vi "MultiChannelFeedback_test_no_before (FPGA).vi"() -> ()   [LabVIEW 2016]
doc: "This VI will read single point values from 4 channels of a R Series board at a specified rate."
uses:
  <vilib>/rvi/Emulation/niFpgaGetClockAttributes.vi
  <vilib>/rvi/Emulation/niFpgaSctlEmulationGetInTimedLoop.vi
  <vilib>/rvi/Emulation/niFpgaEmulationReportErrorSimple.vi
  <vilib>/rvi/Emulation/niFpgaProcessEmulError.vi
  <vilib>/rvi/eio/common/nirviEmuTemplateMethod_errors.vi
  <vilib>/rvi/Emulation/niFpgaCriticalErrorInLSC.vi
  <vilib>/rvi/Memory/Memory_Emulation/nirvimemoryFastEmulation.vi
  <vilib>/rvi/Memory/Memory_Emulation/nirvimemoryEmulation.vi
  <vilib>/rvi/Emulation/niFpgaEmulationIsFPGAContextNoSignature.vi
  <vilib>/rvi/DataTransferAndStorage/Container/Common/niFpgaContainerGetUniqueNameForEmu.vi
  <vilib>/rvi/errors/nirviReportUnexpectedCaseInternalError (U32).vi
  <vilib>/rvi/Memory/Memory_Emulation/niFpgaMemoryEmulationCacheClearOnFirstRun.vi
  <vilib>/rvi/Memory/Memory_Emulation/nirvimemoryEmulationManagerCache_MakeExclusive.vi
  <vilib>/rvi/Memory/Memory_Emulation/niFpgaMemoryEmulationValidateCache.vi
  <vilib>/rvi/Memory/Memory_Emulation/nirvimemoryEmulationManagerCache_InsertValue.vi
  <vilib>/Utility/error.llb/Clear Errors.vi
  <vilib>/rvi/Memory/Memory_Emulation/nirvimemoryEmulationManagerCache_ReleaseExclusive.vi
  <vilib>/rvi/Memory/Memory_Emulation/nirvimemoryEmulationManagerCache_GetValue.vi
  <vilib>/rvi/Memory/Memory_Emulation/nirvimemoryEmulationManagerCache_SetValue.vi
  <vilib>/rvi/Emulation/niFpgaSctlEmulationResourceMgr.vi
  <vilib>/eio/EIONode/EIONode.xnode
  <vilib>/rvi/DataTransferAndStorage/Container/XNode/niFpgaContainer.xnode
  <vilib>/rvi/FXPMathLib/FxpInterpret/XNode/nifxpmath_Interpret.xnode
panel:
  in  "final filter coeff X":i32[](array[numeric])=[-955995012, 2025731616, 1001305, -1023351008, 2092954700, 1034533]
  in  "final filter coeff Y":i32[](array[numeric])=[-955995012, 2025731616, 1001305, -1023351008, 2092954700, 1034533]
  in  "final filter coeff Z":i32[](array[numeric])=[-955995012, 2025731616, 1001305, -1023351008, 2092954700, 1034533]
  in  "LP Coeff Z":i32[](array[numeric])=[1008310688, 32715568]
  in  "LP Coeff X":i32[](array[numeric])=[1008310688, 32715568]
  in  "LP Coeff Y":i32[](array[numeric])=[1008310688, 32715568]
  in  "LP Coeff band X":i32[](array[numeric])=[-955995012, 2025731616, 1001305, -1023351008, 2092954700, 1034533]
  in  "HP Coeff band X":i32[](array[numeric])=[-850883994, 1909449570, 958518847, -975456236, 2033039520, 1020559395]
  in  "dg band X":fxp<+/-,24,12>
  in  "HP Coeff X":i32[](array[numeric])=[946630756, 1010186290]
  out "tot_fb X plot":i16
  in  "DC offset X":i16
  out "fb X plot":i16
  in  "ig X":fxp<+/-,24,6>
  in  "Lower lim X":fxp<+/-,16,16>
  in  "Upper lim X":fxp<+/-,16,16>
  in  "dg X":fxp<+/-,24,12>
  in  "pg X":fxp<+/-,24,12>
  out "AI X plot":i16
  in  "X Setpoint":i16
  in  "LP Coeff band Y":i32[](array[numeric])=[-955995012, 2025731616, 1001305, -1023351008, 2092954700, 1034533]
  in  "HP Coeff band Y":i32[](array[numeric])=[-850883994, 1909449570, 958518847, -975456236, 2033039520, 1020559395]
  in  "dg band Y":fxp<+/-,24,12>
  in  "HP Coeff Y":i32[](array[numeric])=[946630756, 1010186290]
  out "tot_fb Y plot":i16
  in  "DC offset Y":i16
  out "fb Y plot":i16
  in  "ig Y":fxp<+/-,24,6>
  in  "Lower lim Y":fxp<+/-,16,16>
  in  "Upper lim Y":fxp<+/-,16,16>
  in  "dg Y":fxp<+/-,24,12>
  in  "pg Y":fxp<+/-,24,12>
  out "AI Y plot":i16
  in  "Y Setpoint":i16
  in  "EOM_offset":i16
  in  "EOM_seed":u32=4294967295 caption="seed"
  in  "EOM reset":bool caption="reset"
  in  "EOM_threshold":i16
  in  "EOM_amplitude":i16
  in  "LP Coeff band Z":i32[](array[numeric])=[-955995012, 2025731616, 1001305, -1023351008, 2092954700, 1034533]
  in  "HP Coeff band Z":i32[](array[numeric])=[-850883994, 1909449570, 958518847, -975456236, 2033039520, 1020559395]
  in  "dg band Z":fxp<+/-,24,12>
  in  "data_buffer3":i16
  in  "Arb gain (ch2)":fxp<+/-,24,12>=0.5 caption="RMS"
  in  "HP Coeff Z":i32[](array[numeric])=[946630756, 1010186290]
  out "tot_fb Z plot":i16
  in  "DC offset Z":i16
  out "fb Z plot":i16
  in  "ig Z":fxp<+/-,24,6>
  out "written_address":u32
  in  "ready_to_write":bool
  in  "Arb steps per cycle":u16
  in  "data_buffer2":i16
  in  "data_buffer_1":i16
  in  "write_address":u16
  in  "Arb gain (ch1)":fxp<+/-,24,12>=0.5 caption="RMS"
  in  "Arb gain (ch0)":fxp<+/-,24,12>=0.5 caption="RMS"
  in  "Lower lim Z":fxp<+/-,16,16>
  in  "Upper lim Z":fxp<+/-,16,16>
  in  "dg Z":fxp<+/-,24,12>
  in  "pg Z":fxp<+/-,24,12>
  out "AI Z plot":i16
  in  "Z Setpoint":i16
  in  "Count(uSec)":u32
  out "FPGA Error Out":errorcluster
  in  "Stop":bool
  # "test"
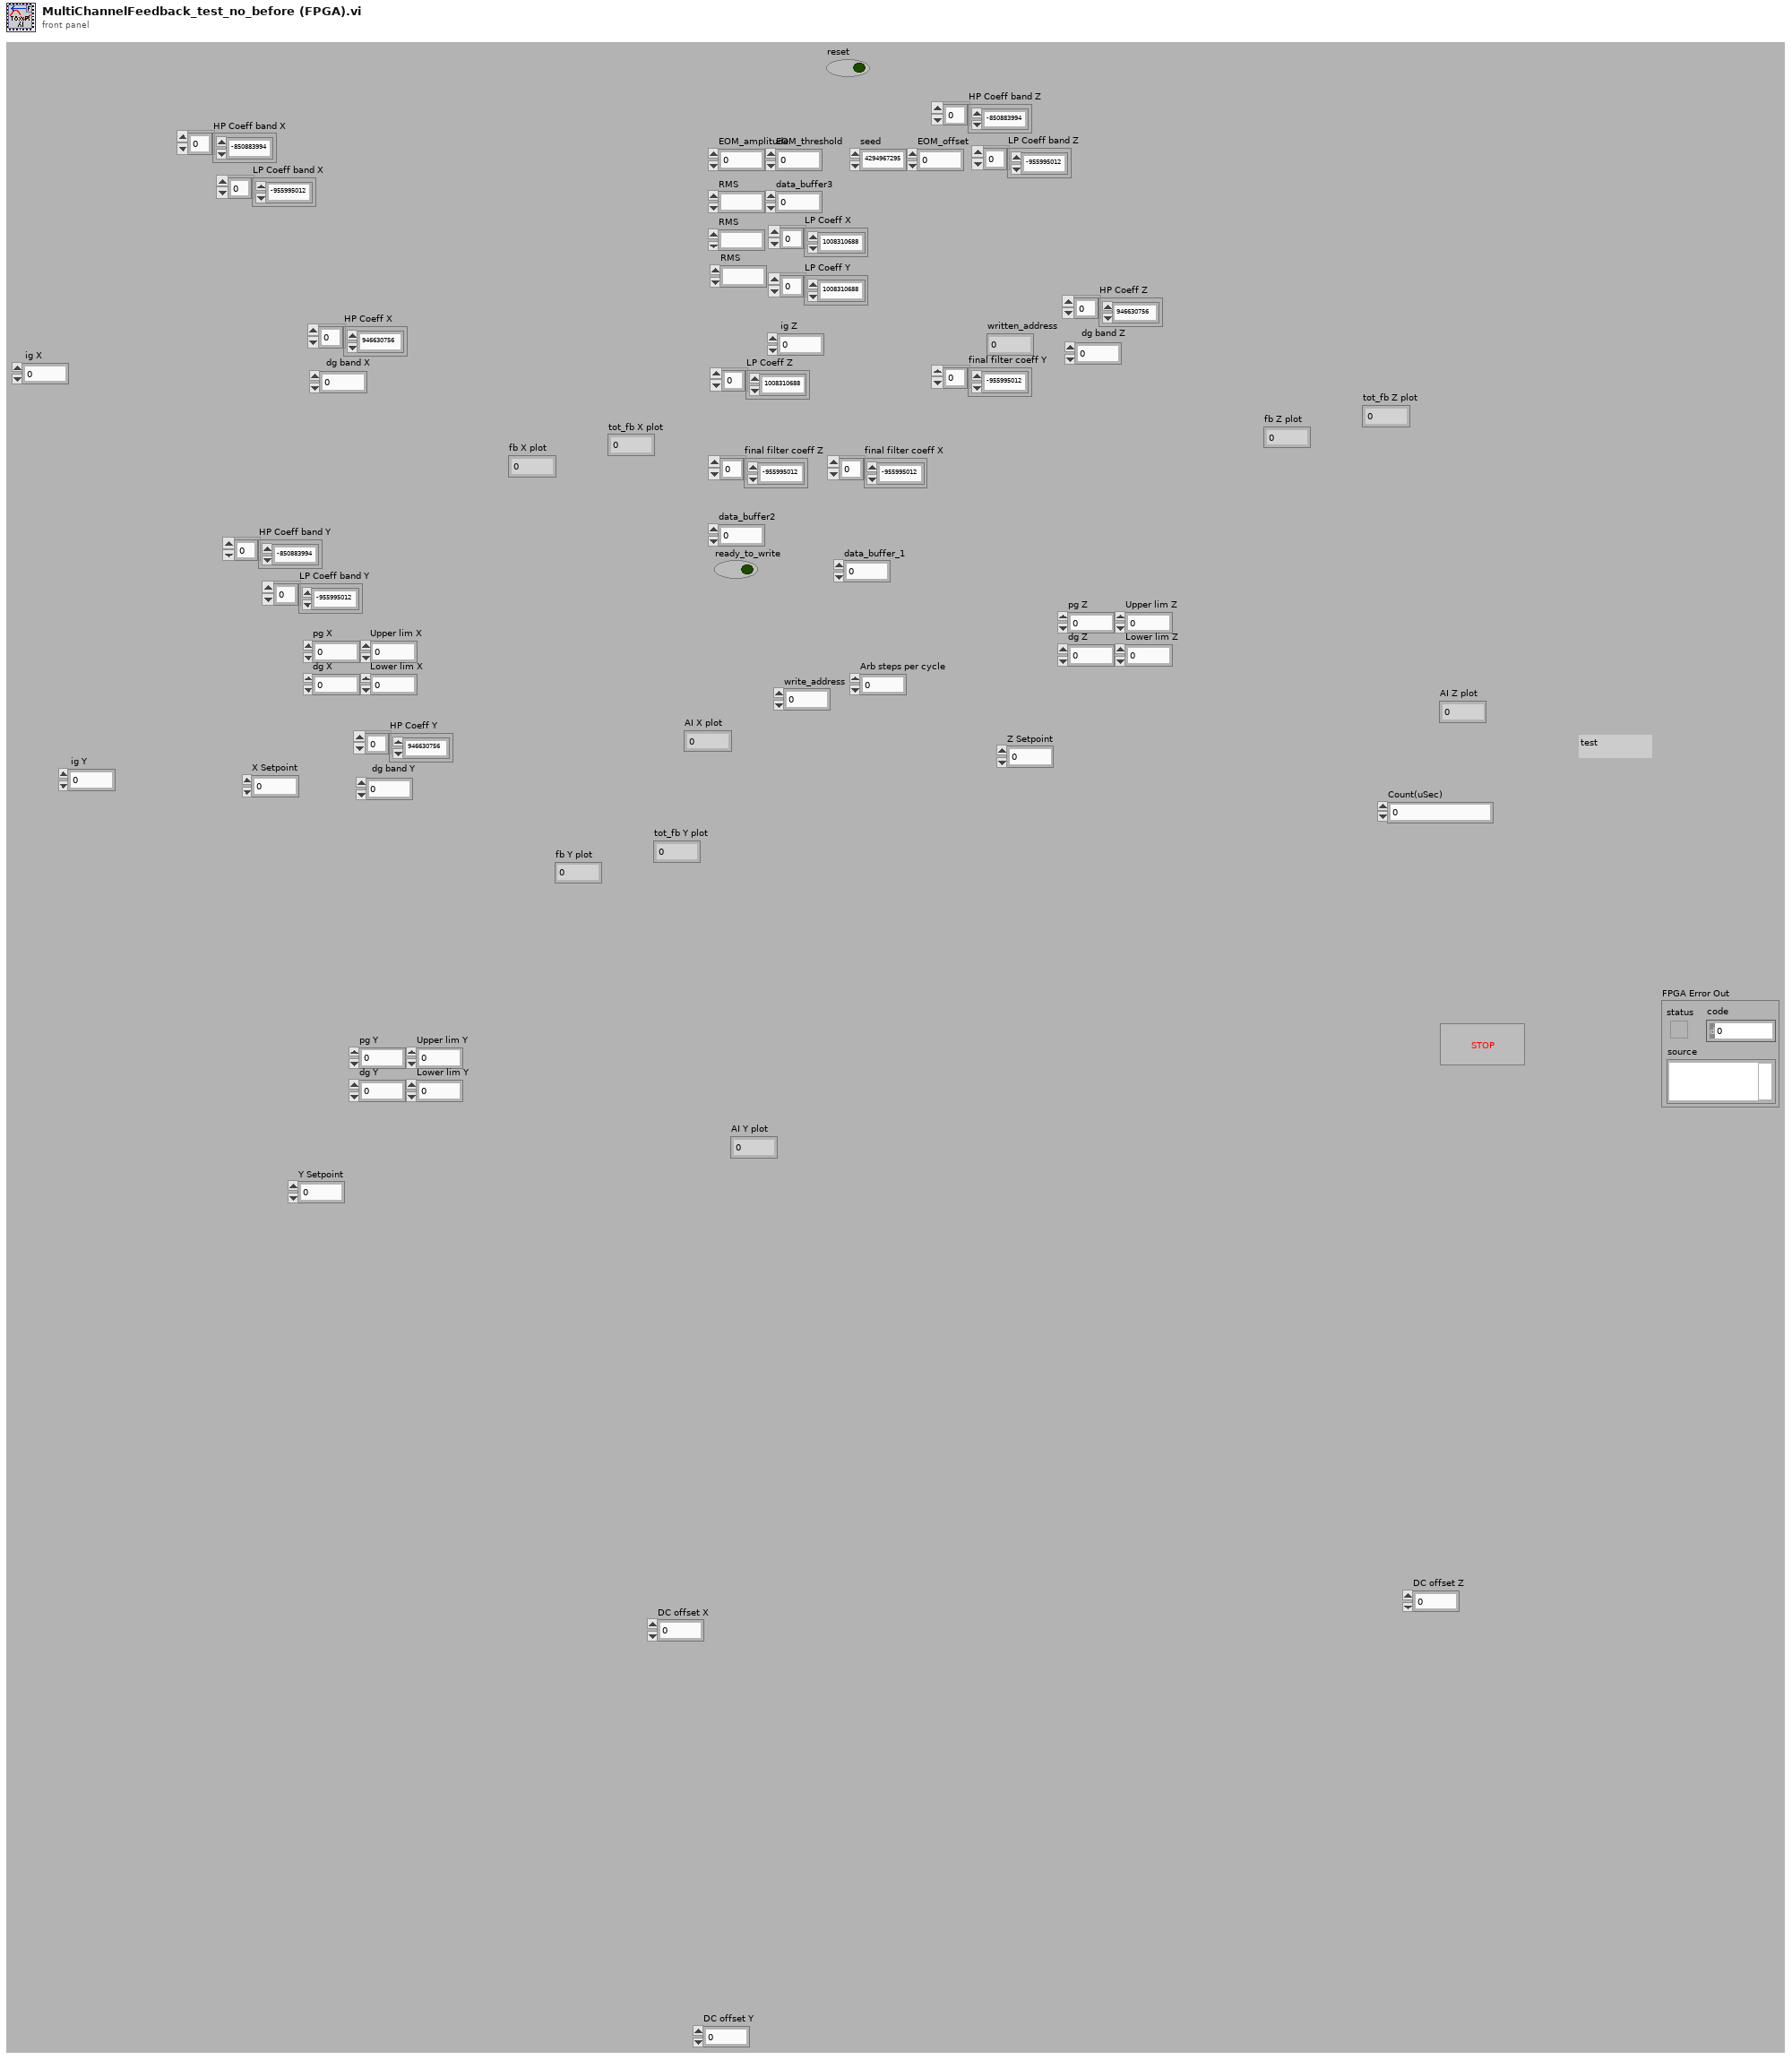
[diagram p1: front panel]
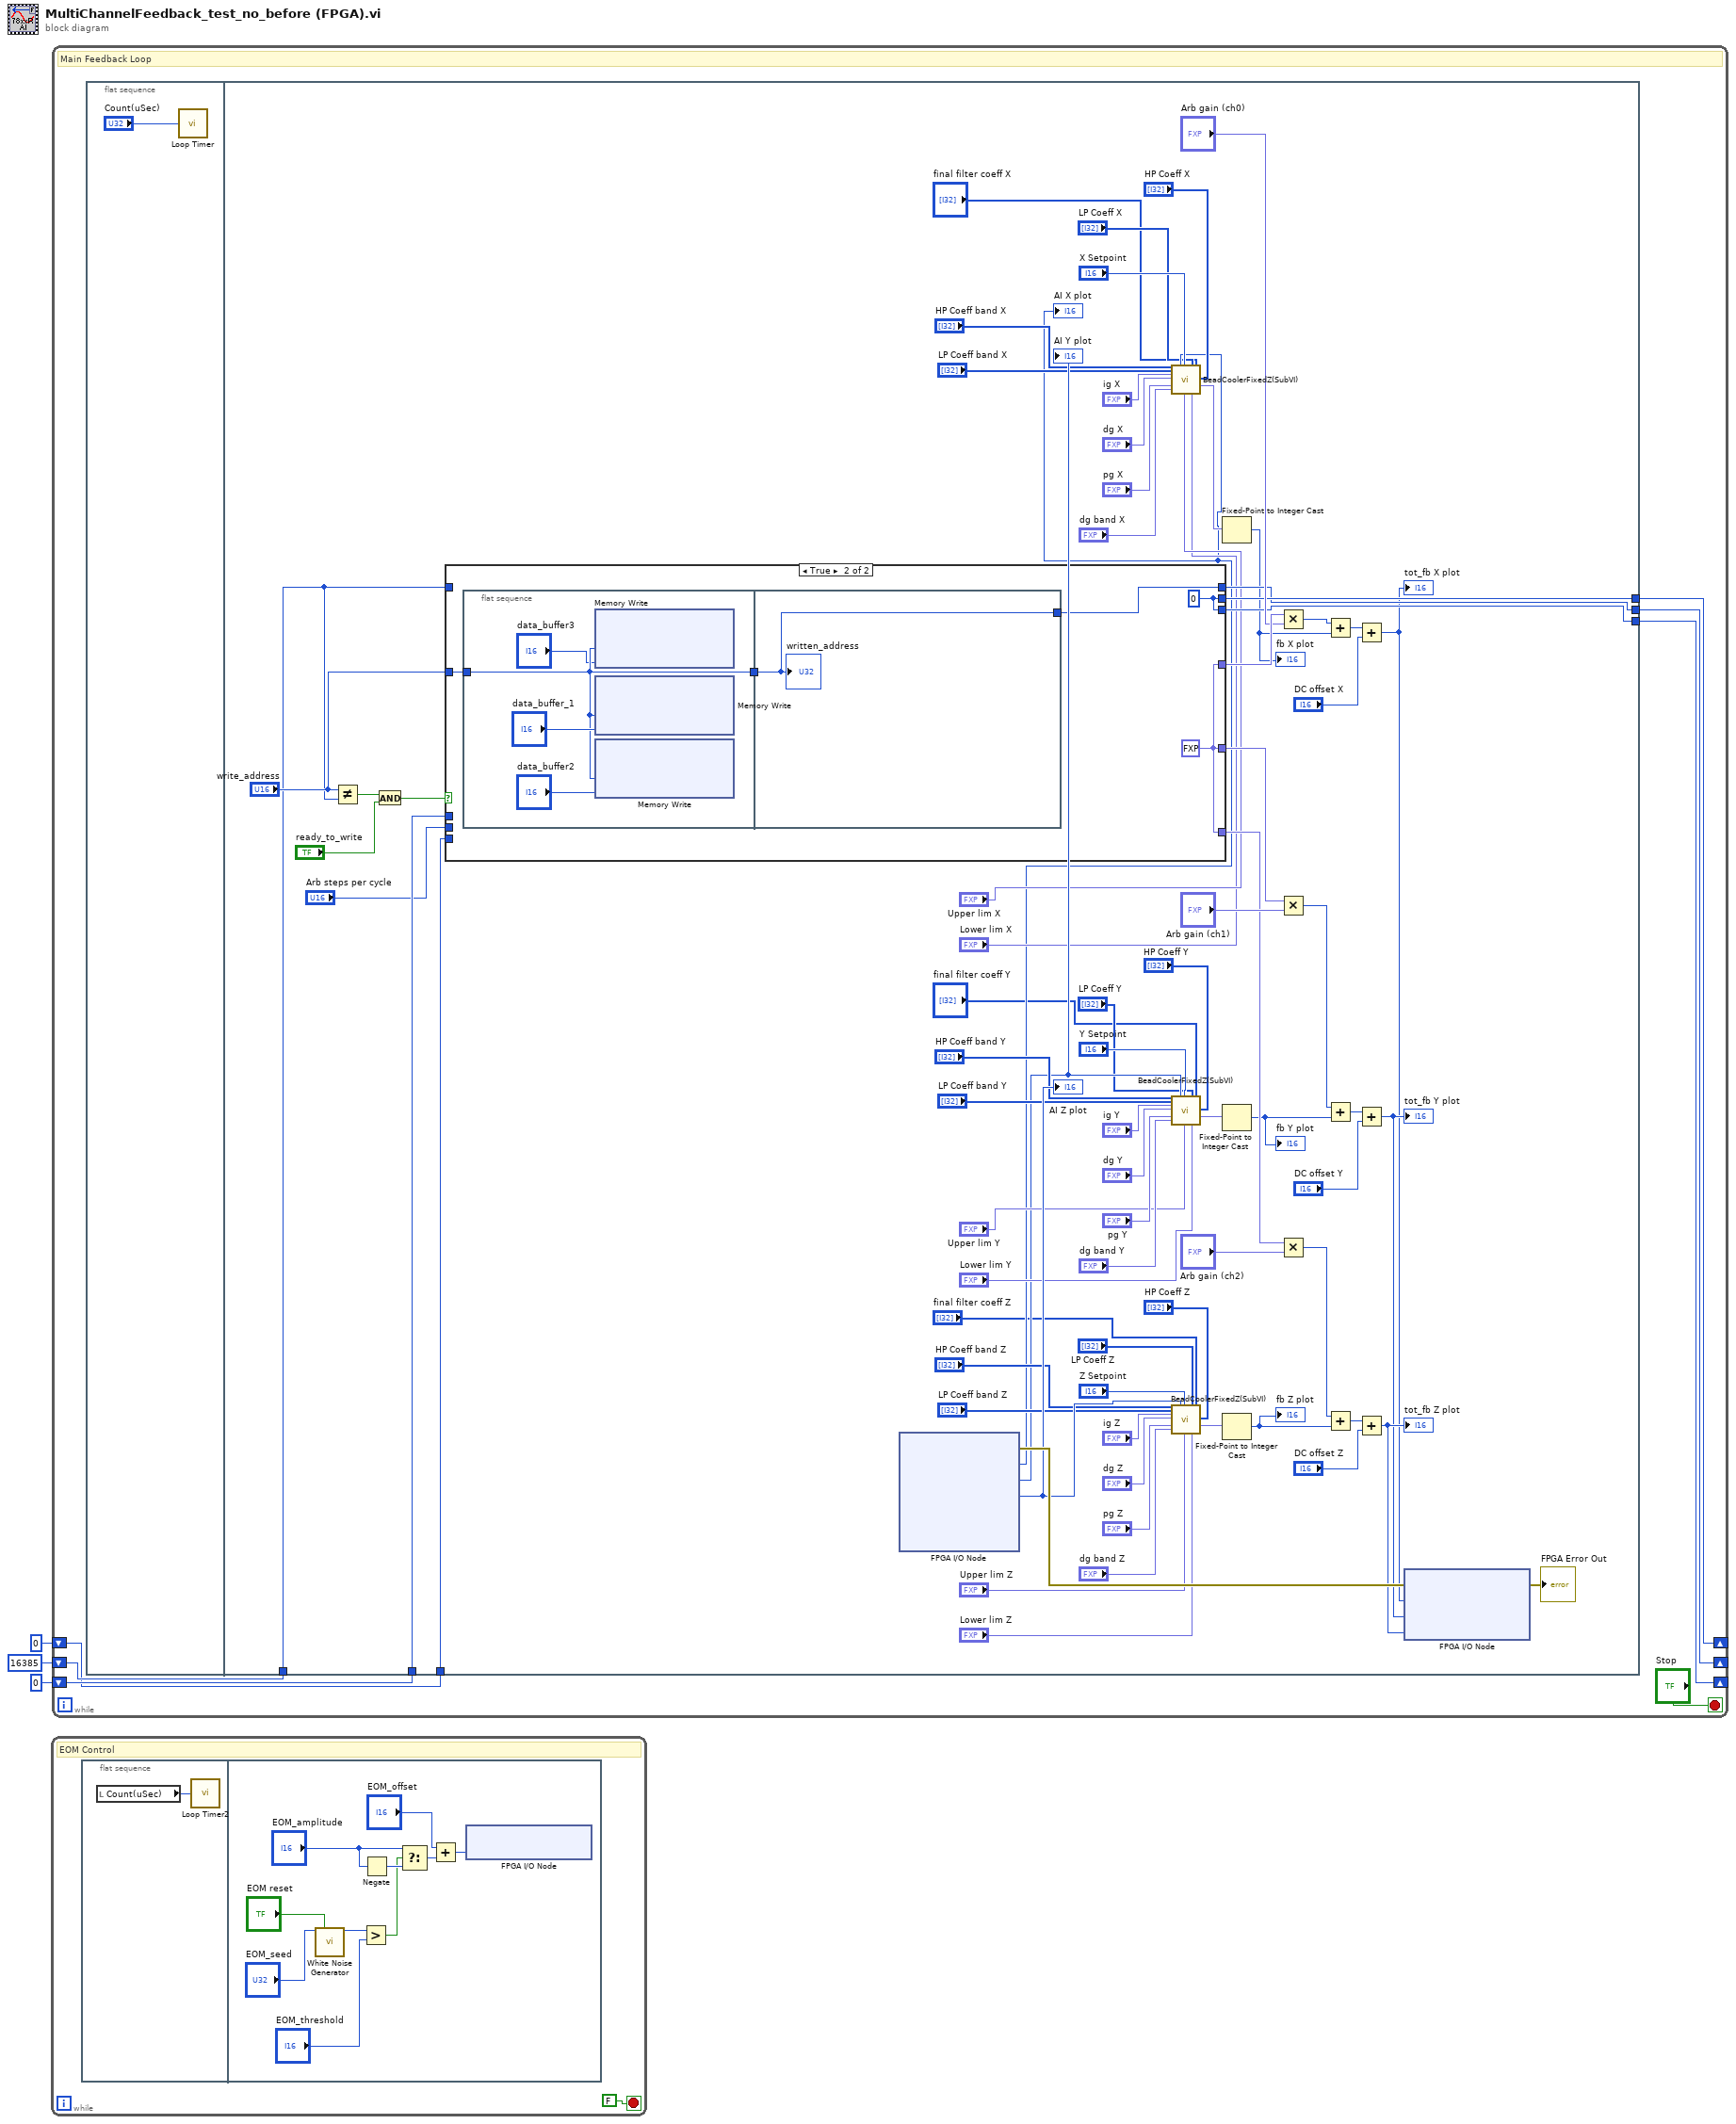
[diagram p0: block diagram]
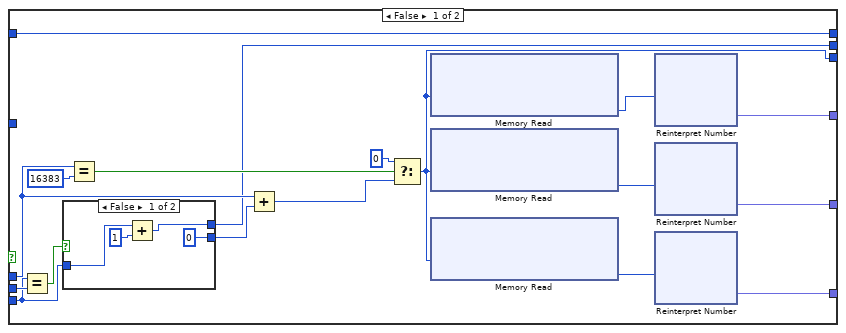
[diagram p2: hidden frame]
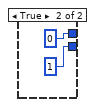
[diagram p3: hidden frame]
diagram:
  n1 = while {
    stop <- FALSE stop-if-true
    # "EOM Control"
    n2 = flat-sequence {
      frame #0 {
        n3 = local read "Count(uSec)"() -> (w5:u32)
        n4 = call "Loop Timer2"("Count(uSec)"=w5) -> ()  [unwired: 1 out]
      }
      frame #1 {
        n5 = call "White Noise Generator"("seed"="EOM_seed", "reset"="EOM reset") -> ("white noise out"=w7:i16)  [unwired: 13 in]
        n6 = Greater?(x=w7, y="EOM_threshold") -> (0:w9:bool)
        n7 = Negate(x="EOM_amplitude") -> (-x=w11:i16)
        n8 = Select(t="EOM_amplitude", s=w9, f=w11) -> (s? t:f=w14:i16)
        n9 = Add(x="EOM_offset", y=w14) -> (x+y=w6:i16)
        n10 = xnode "FPGA I/O Node"("Connector0/AO3"=w6) -> ()  [unwired: 1 in, 1 out]
      }
    }
  }
  n11 = while {
    shift-right: [w21] -> _
    shift-left: u16 0 ("t") -> [w20]
    shift-right: [w19] -> _
    shift-left: u16 0 ("t") -> [w16]
    shift-right: [w18] -> _
    shift-left: u32 16385 ("write_address") -> [w17]
    stop <- "Stop" stop-if-true
    # "Main Feedback Loop"
    n12 = flat-sequence {
      tunnel: [w92] -> w21
      tunnel: w20 -> [w91]
      tunnel: [w89] -> w19
      tunnel: w16 -> [w88]
      tunnel: [w87] -> w18
      tunnel: w17 -> [w80]
      frame #0 {
        n13 = call "Loop Timer"("Count(uSec)"="Count(uSec)") -> ()  [unwired: 1 out]
      }
      frame #1 {
        n14 = Not Equal?(x="write_address", y=w80) -> (x != y?=w84:bool)
        n15 = And(x=w84, y="ready_to_write") -> (x .and. y?=w85:bool)
        n16 = case shown="True" w85 {
          tunnel: [w116 w124] -> w94
          tunnel: [w101 w128] -> w92
          tunnel: w91 -> [w109 _]
          tunnel: [w110 w124] -> w82
          tunnel: "Arb steps per cycle" -> [w108 _]
          tunnel: [w103 w128] -> w89
          tunnel: w88 -> [w104 _]
          tunnel: [w107 w126] -> w87
          tunnel: w80 -> [w107 _]
          tunnel: "write_address" -> [_ w125]
          tunnel: [w100 w124] -> w72
          frame False {
            n17 = Equal?(x=w104, y=w108) -> (x = y?=w106:bool)
            n18 = case shown="False" w106 {
              tunnel: [u16 0 ("y") u16 1 ("y")] -> w105
              tunnel: w104 -> [w120 _]
              tunnel: [w118 u16 0] -> w103
              frame False {
                n19 = Add(x=w120, y=u16 1) -> (x+y=w118:u16)
              }
              frame True {
              }
            }
            n20 = Equal?(x=w109, y=u16 16383) -> (x = y?=w114:bool)
            n21 = Add(x=w109, y=w105) -> (x+y=w112:u16)
            n22 = Select(t=u16 0, s=w114, f=w112) -> (s? t:f=w101:u16)
            n23 = xnode ("Memory Read")("Address"=w101) -> ("Data"=w117:i16)  [unwired: 1 in, 1 out]
            n24 = xnode ("Memory Read")("Address"=w101) -> ("Data"=w111:i16)  [unwired: 1 in, 1 out]
            n25 = xnode ("Memory Read")("Address"=w101) -> ("Data"=w102:i16)  [unwired: 1 in, 1 out]
            n26 = xnode "Reinterpret Number"("x"=w117) -> ("y"=w116:fxp<+/-,16,16>)
            n27 = xnode "Reinterpret Number"("x"=w111) -> ("y"=w110:fxp<+/-,16,16>)
            n28 = xnode "Reinterpret Number"("x"=w102) -> ("y"=w100:fxp<+/-,16,16>)
          }
          frame True {
            w128 = u16 0
            w124 = fxp<+/-,16,16> 0.0 ("y")
            n29 = flat-sequence {
              tunnel: [w130] -> w127
              tunnel: w125 -> [w130]
              tunnel: w127 -> [w133]
              tunnel: [w133] -> w126
              frame #0 {
                n30 = xnode ("Memory Write")("Address"=w130, "Data"="data_buffer3") -> ()  [unwired: 1 in, 1 out]
                n31 = xnode ("Memory Write")("Address"=w130, "Data"="data_buffer_1") -> ()  [unwired: 1 in, 1 out]
                n32 = xnode ("Memory Write")("Address"=w130, "Data"="data_buffer2") -> ()  [unwired: 1 in, 1 out]
              }
              frame #1 {
                "written_address" <- w133
              }
            }
          }
        }
        n33 = xnode "FPGA I/O Node"() -> ("error out"=w99:errorcluster, "Connector0/AI0"=w40:i16, "Connector0/AI1"=w54:i16, "Connector0/AI2"=w78:i16)  [unwired: 7 in, 9 out]
        "AI Z plot" <- w78
        "AI Y plot" <- w54
        "AI X plot" <- w40
        n34 = call "BeadCoolerFixedZ(SubVI).vi"("hp coeff band"="HP Coeff band X", "lp coeff band"="LP Coeff band X", "ig"="ig X", "dg"="dg X", "pg"="pg X", "dg band"="dg band X", "AI0"=w40, "Dc Pos"="X Setpoint", "Upper lim"="Upper lim X", "lp coeff"="LP Coeff X", "Lower lim"="Lower lim X", "final filter coeff"="final filter coeff X", "hp coeff"="HP Coeff X") -> ("Output"=w46:fxp<+/-,16,16>)  [unwired: 14 in]
        n35 = call "BeadCoolerFixedZ(SubVI).vi"("hp coeff band"="HP Coeff band Y", "lp coeff band"="LP Coeff band Y", "ig"="ig Y", "dg"="dg Y", "pg"="pg Y", "dg band"="dg band Y", "AI0"=w54, "Dc Pos"="Y Setpoint", "Upper lim"="Upper lim Y", "lp coeff"="LP Coeff Y", "Lower lim"="Lower lim Y", "final filter coeff"="final filter coeff Y", "hp coeff"="HP Coeff Y") -> ("Output"=w60:fxp<+/-,16,16>)  [unwired: 14 in]
        n36 = call "BeadCoolerFixedZ(SubVI).vi"("hp coeff band"="HP Coeff band Z", "lp coeff band"="LP Coeff band Z", "ig"="ig Z", "dg"="dg Z", "pg"="pg Z", "dg band"="dg band Z", "AI0"=w78, "Dc Pos"="Z Setpoint", "Upper lim"="Upper lim Z", "lp coeff"="LP Coeff Z", "Lower lim"="Lower lim Z", "final filter coeff"="final filter coeff Z", "hp coeff"="HP Coeff Z") -> ("Output"=w74:fxp<+/-,16,16>)  [unwired: 14 in]
        n37 = Fixed-Point to Integer Cast(1:w46) -> (0:w26:i16)
        "fb X plot" <- w26
        n38 = Fixed-Point to Integer Cast(1:w60) -> (0:w25:i16)
        "fb Y plot" <- w25
        n39 = Fixed-Point to Integer Cast(1:w74) -> (0:w24:i16)
        "fb Z plot" <- w24
        n40 = Multiply(x=w94, y="Arb gain (ch0)") -> (x*y=w32:i16)
        n41 = Multiply(x=w82, y="Arb gain (ch1)") -> (x*y=w31:i16)
        n42 = Multiply(x=w72, y="Arb gain (ch2)") -> (x*y=w30:i16)
        n43 = Add(x=w32, y=w26) -> (x+y=w29:i16)
        n44 = Add(x=w31, y=w25) -> (x+y=w28:i16)
        n45 = Add(x=w30, y=w24) -> (x+y=w27:i16)
        n46 = Add(x=w29, y="DC offset X") -> (x+y=w39:i16)
        "tot_fb X plot" <- w39
        n47 = Add(x=w28, y="DC offset Y") -> (x+y=w53:i16)
        "tot_fb Y plot" <- w53
        n48 = Add(x=w27, y="DC offset Z") -> (x+y=w76:i16)
        "tot_fb Z plot" <- w76
        n49 = xnode "FPGA I/O Node"("error in"=w99, "Connector0/AO0"=w39, "Connector0/AO1"=w53, "Connector0/AO2"=w76) -> ("error out"=→"FPGA Error Out":errorcluster)  [unwired: 3 in, 3 out]
      }
    }
  }
